vi "User Interface.vi"(8 "error in (no error)":errorcluster, 11 "User Interface in":refnum<class "User Interface.lvclass">) -> (0 "error out":errorcluster, 3 "User Interface out":refnum<class "User Interface.lvclass">)   [LabVIEW 2017, in "DSF Core.lvlib" / "Core Group User Interface.lvclass"]
uses:
  Core Group User Interface.lvclass
  User Interface.lvclass
  Configuration/Base/Group/Group Configuration.lvclass
  C:/Git/DSF/Core/Classes/Configuration/Configuration.lvclass
  Configuration/Configuration.lvclass
panel:
  in  "Enable Conversion":bool
  in  "Timeout Behavior":enum16{"Increment Late Count", "Throw Error"}(ring)
  in  "Offset":u64
  in  "Decimation":u64
  in  "Priority":u64
  in  "Direction":enum16{"Tx", "Rx"}(ring)
  in  "Name":string
  out "Data Version":string
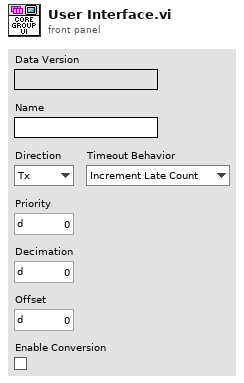
[diagram p1: front panel]
types:
  T1 = typedef "DSF Core.lvlib/Group Configuration.lvclass/Core Group Configuration.ctl" = cluster{"name":string, "direction":T2, "cycle timing":T3, "timeout behavior":T4, "enable conversion":bool}
  T2 = typedef "DSF Core.lvlib/DSF Direction.ctl" = enum8{"Tx", "Rx"}
  T3 = typedef "DSF Core.lvlib/DSF Timing Info.ctl" = cluster{"priority":u64, "decimation":u64, "offset":u64}
  T4 = typedef "DSF Core.lvlib/DSF Timeout Behavior.ctl" = enum8{"Increment Late Count", "Throw Error"}
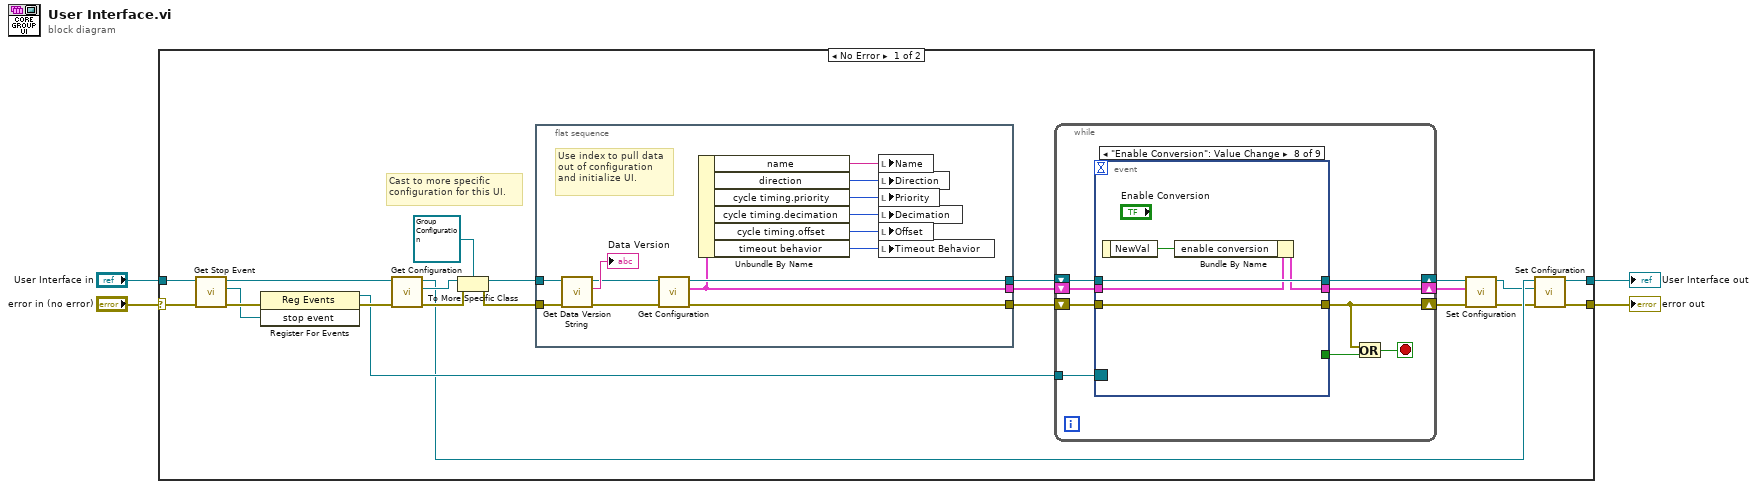
[diagram p0: block diagram]
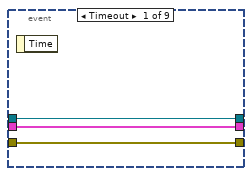
[diagram p2: hidden frame]
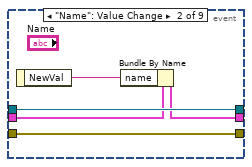
[diagram p3: hidden frame]
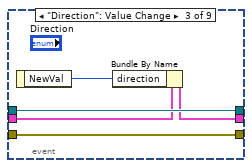
[diagram p4: hidden frame]
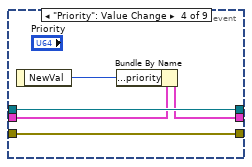
[diagram p5: hidden frame]
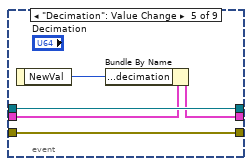
[diagram p6: hidden frame]
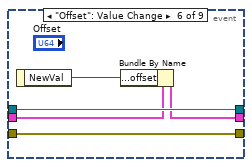
[diagram p7: hidden frame]
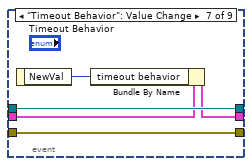
[diagram p8: hidden frame]
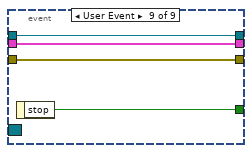
[diagram p9: hidden frame]
diagram:
  n1 = case shown="No Error" "error in (no error)" {
    selector: "error in (no error)" -> [w22 w94]
    tunnel: [w13 w94] -> w4
    tunnel: "User Interface in" -> [w21 w93]
    tunnel: [w12 w93] -> w1
    frame No Error {
      # "Cast to more specific configuration for this UI."
      n2 = call "Get Stop Event.vi"("error in (no error)"=w22, "User Interface in"=w21) -> ("error out"=w20:errorcluster, "stop event"=w19:refnum<user-event>, "User Interface out"=w16:refnum<class "User Interface.lvclass">)  [unwired: 7 in]
      n3 = register-events(error in=w20, w19) -> (reference out=w15:refnum<event-registration>, error out=w18:errorcluster)  [unwired: 1 in]
      n4 = call "Get Configuration.vi"("error in (no error)"=w18, "User Interface in"=w16) -> ("error out"=w17:errorcluster, "configuration"=w14:refnum<class "Configuration.lvclass">, "User Interface out"=w11:refnum<class "User Interface.lvclass">)  [unwired: 7 in]
      n5 = To More Specific Class(target class=refnum<class "Group Configuration.lvclass"> refnum ("DSF Core.lvlib:Group Configuration.lvclass"), reference=w14, error in=w17) -> (specific class reference=w27:refnum<class "Group Configuration.lvclass">, error out=w24:errorcluster)
      n6 = flat-sequence {
        tunnel: [w30] -> w25
        tunnel: w24 -> [w41]
        tunnel: w27 -> [w40]
        tunnel: [w29] -> w26
        tunnel: [w28] -> w23
        frame #0 {
          # "Use index to pull data out of configuration and initialize UI."
          n7 = call "Get Data Version String.vi"("error in (no error)"=w41, "Configuration in"=w40) -> ("error out"=w31:errorcluster, "data version"=→"Data Version":string, "Configuration out"=w32:refnum<class "Group Configuration.lvclass">)  [unwired: 7 in]
          n8 = call "Get Configuration.vi"("error in (no error)"=w31, "Core Groups Configuration in"=w32) -> ("error out"=w30:errorcluster, "configuration"=w28:T1, "Core Groups Configuration out"=w29:refnum<class "Group Configuration.lvclass">)  [unwired: 7 in]
          n9 = Unbundle By Name(w28) -> ("name"=w38:string, "direction"=w37:T2, "cycle timing.priority"=w36:u64, "cycle timing.decimation"=w35:u64, "cycle timing.offset"=w34:u64, "timeout behavior"=w33:T4)
          n10 = local write "Name"(w38) -> ()
          n11 = local write "Direction"(w37) -> ()
          n12 = local write "Priority"(w36) -> ()
          n13 = local write "Decimation"(w35) -> ()
          n14 = local write "Offset"(w34) -> ()
          n15 = local write "Timeout Behavior"(w33) -> ()
        }
      }
      n16 = while {
        tunnel: w15 -> [w50]
        shift-right: [w48] -> w9
        shift-left: w25 -> [w49]
        shift-right: [w44] -> w7
        shift-left: w26 -> [w45]
        shift-right: [w42] -> w5
        shift-left: w23 -> [w43]
        stop <- w47 stop-if-true
        n17 = event shown="[7] \"Enable Conversion\": Value Change" {
          selector: w50 -> [_ _ _ _ _ _ _ _ _]
          dyn-events: _ -> [_ _ _ _ _ _ _ _ _]
          timeout: _ -> [_ _ _ _ _ _ _ _ _]
          tunnel: [_ _ _ _ _ _ _ _ w90] -> w46
          tunnel: w49 -> [w53 w58 w63 w68 w73 w78 w83 w88 w92]
          tunnel: [w53 w58 w63 w68 w73 w78 w83 w88 w92] -> w48
          tunnel: w45 -> [w52 w57 w62 w67 w72 w77 w82 w87 w91]
          tunnel: [w52 w57 w62 w67 w72 w77 w82 w87 w91] -> w44
          tunnel: w43 -> [w51 w56 w61 w66 w71 w76 w81 w86 w89]
          tunnel: [w51 w55 w60 w65 w70 w75 w80 w85 w89] -> w42
          event Timeout {
            n18 = event-data() -> ()  [unwired: 1 in, 1 out]
          }
          event "Name": Value Change {
            n19 = event-data() -> ("NewVal"=w54:string)  [unwired: 1 in]
            n20 = Bundle By Name(cluster=w56, "name"=w54) -> (w55:T1)
          }
          event "Direction": Value Change {
            n21 = event-data() -> ("NewVal"=w59:enum16{"Tx", "Rx"})  [unwired: 1 in]
            n22 = Bundle By Name(cluster=w61, "direction"=w59) -> (w60:T1)
          }
          event "Priority": Value Change {
            n23 = event-data() -> ("NewVal"=w64:u64)  [unwired: 1 in]
            n24 = Bundle By Name(cluster=w66, "cycle timing.priority"=w64) -> (w65:T1)
          }
          event "Decimation": Value Change {
            n25 = event-data() -> ("NewVal"=w69:u64)  [unwired: 1 in]
            n26 = Bundle By Name(cluster=w71, "cycle timing.decimation"=w69) -> (w70:T1)
          }
          event "Offset": Value Change {
            n27 = event-data() -> ("NewVal"=w74:u64)  [unwired: 1 in]
            n28 = Bundle By Name(cluster=w76, "cycle timing.offset"=w74) -> (w75:T1)
          }
          event "Timeout Behavior": Value Change {
            n29 = event-data() -> ("NewVal"=w79:enum16{"Increment Late Count", "Throw Error"})  [unwired: 1 in]
            n30 = Bundle By Name(cluster=w81, "timeout behavior"=w79) -> (w80:T1)
          }
          event "Enable Conversion": Value Change {
            n31 = event-data() -> ("NewVal"=w84:bool)  [unwired: 1 in]
            n32 = Bundle By Name(cluster=w86, "enable conversion"=w84) -> (w85:T1)
          }
          event User Event {
            n33 = event-data() -> ("stop"=w90:bool)  [unwired: 1 in]
          }
        }
        n34 = Or(x=w48, y=w46) -> (x .or. y?=w47:bool)
      }
      n35 = call "Set Configuration.vi"("error in (no error)"=w9, "configuration"=w5, "Core Groups Configuration in"=w7) -> ("error out"=w8:errorcluster, "Core Groups Configuration out"=w6:refnum<class "Group Configuration.lvclass">)  [unwired: 7 in]
      n36 = call "Set Configuration.vi"("error in (no error)"=w8, "configuration"=w6, "User Interface in"=w11) -> ("error out"=w13:errorcluster, "User Interface out"=w12:refnum<class "User Interface.lvclass">)  [unwired: 7 in]
    }
    frame Error {
    }
  }
  "error out" <- w4
  "User Interface out" <- w1
